vi "CheckIfFileExist-SubVI.vi"(11 "Path in":refnum<vi>) -> ()   [LabVIEW 2019]
uses:
  <vilib>/Utility/file.llb/Write Delimited Spreadsheet (string).vi
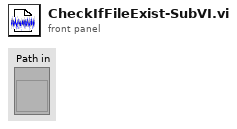
[diagram p1: front panel]
types:
  T1 = enum16{"open", "replace", "create", "open or create", "replace or create", "replace or create with confirmation"}
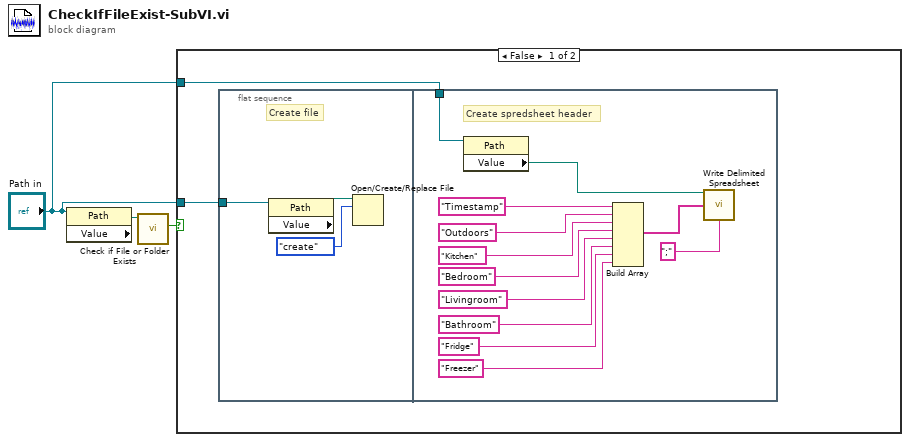
[diagram p0: block diagram]
diagram:
  n1 = property class="Path"(reference="Path in") -> ("Value"=w3:path)  [unwired: 1 in, 2 out]
  n2 = call <vilib>:"Check if File or Folder Exists.vi"("path"=w3) -> ("file or folder exists?"=w2:bool)  [unwired: 8 in, 2 out]
  n3 = case shown="False" w2 {
    tunnel: "Path in" -> [w5 _]
    tunnel: "Path in" -> [w4 _]
    frame False {
      n4 = flat-sequence {
        tunnel: w5 -> [w6]
        tunnel: w4 -> [w17]
        frame #0 {
          # "Create file"
          n5 = property class="Path"(reference=w6) -> ("Value"=w8:path)  [unwired: 1 in, 2 out]
          n6 = Open/Create/Replace File(file path (use dialog)=w8, operation (0:open)=T1."create") -> ()  [unwired: 4 in, 3 out]
        }
        frame #1 {
          # "Create spredsheet header"
          n7 = property class="Path"(reference=w17) -> ("Value"=w18:path)  [unwired: 1 in, 2 out]
          n8 = Build Array("Timestamp", "Outdoors", "Kitchen", "Bedroom", "Livingroom", "Bathroom", "Fridge", "Freezer") -> (w20:string[])
          n9 = call-poly <vilib>:"Write Delimited Spreadsheet.vi"("file path (dialog if empty)"=w18, "1D data"=w20, "delimiter (\\t)"=";" ("delimiter (\\t)")) -> ()  [unwired: 11 in, 2 out]
        }
      }
    }
    frame True {
    }
  }
